vi "Main.vi"(10 "JQMHStartup.lvclass":refnum<class "RQMHStartup.lvclass">, 11 "TesterModule in":refnum<class "Watchdog.lvclass">) -> ()   [LabVIEW 2024, in "Watchdog.lvclass"]
uses:
  Watchdog.lvclass
  Startup/RQMHStartup.lvclass
  Watchdog.lvclass/Watchdog.ctl
  Shared/RQMHShared.lvlib
  ModuleCore/RQMHModule.lvclass
panel:
  out "error out":errorcluster
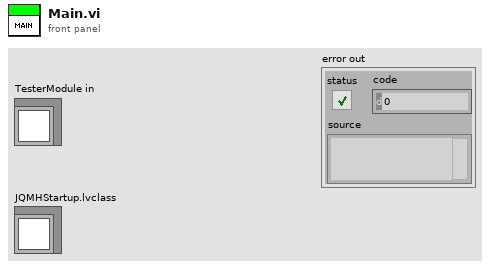
[diagram p1: front panel]
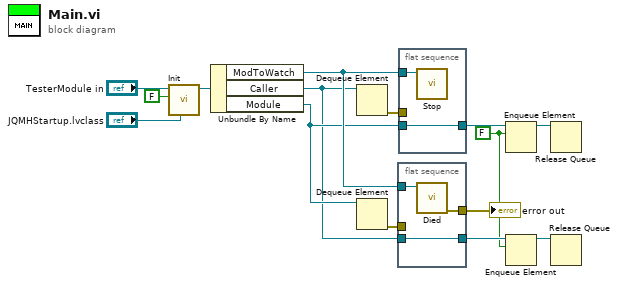
[diagram p0: block diagram]
diagram:
  w4 = FALSE ("element")
  n1 = call "Init.vi"("JQMHStartup.lvclass"="JQMHStartup.lvclass", "Declare? (T)"=FALSE, "JQMHCore.lvclass"="TesterModule in") -> ("JQMHCore out"=w14:refnum<class "Watchdog.lvclass">)  [unwired: 3 in, 5 out]
  n2 = Unbundle By Name(w14) -> ("ModToWatch"=w11:refnum<class "RQMHModule.lvclass">, "Caller"=w5:refnum<queue>, "Module"=w10:refnum<queue>)
  n3 = Dequeue Element(queue=w5) -> (error out=w13:errorcluster)  [unwired: 2 in, 3 out]
  n4 = Dequeue Element(queue=w10) -> (error out=w12:errorcluster)  [unwired: 2 in, 3 out]
  n5 = flat-sequence {
    tunnel: w11 -> [w18]
    tunnel: w12 -> [_]
    tunnel: [w17] -> w6
    tunnel: w5 -> [w17]
    tunnel: [w16] -> w3
    frame #0 {
      n6 = call "Died.vi"("JQMHModule in"=w18) -> ("error out"=w16:errorcluster)  [unwired: 9 in, 1 out]
    }
  }
  n7 = flat-sequence {
    tunnel: w11 -> [w20]
    tunnel: w13 -> [_]
    tunnel: w10 -> [w19]
    tunnel: [w19] -> w9
    frame #0 {
      n8 = call "Stop.vi"("JQMHCore in"=w20) -> ()  [unwired: 10 in, 1 out]
    }
  }
  n9 = Enqueue Element(queue=w9, element=w4) -> (queue out=w8:refnum<queue>)  [unwired: 2 in, 2 out]
  n10 = Enqueue Element(queue=w6, element=w4) -> (queue out=w7:refnum<queue>)  [unwired: 2 in, 2 out]
  n11 = Release Queue(queue=w8) -> ()  [unwired: 2 in, 3 out]
  n12 = Release Queue(queue=w7) -> ()  [unwired: 2 in, 3 out]
  "error out" <- w3
